vi "Problem 3.vi"(11 "Number to Factor":u64=600851475143) -> (2 "List of Factors":u64[](array[numeric]), 3 "Largest Factor":u64=600851475143)   [LabVIEW 2013, in "Problem 3.lvlib"]
uses:
  Problem 3.lvlib
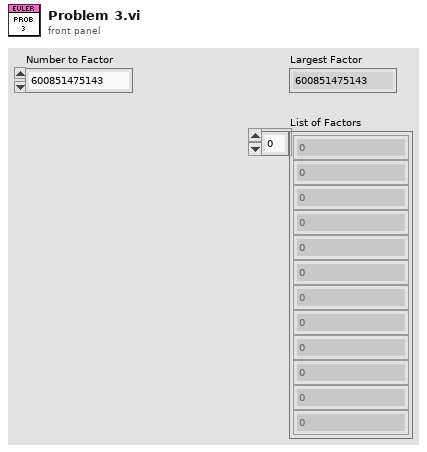
[diagram p1: front panel]
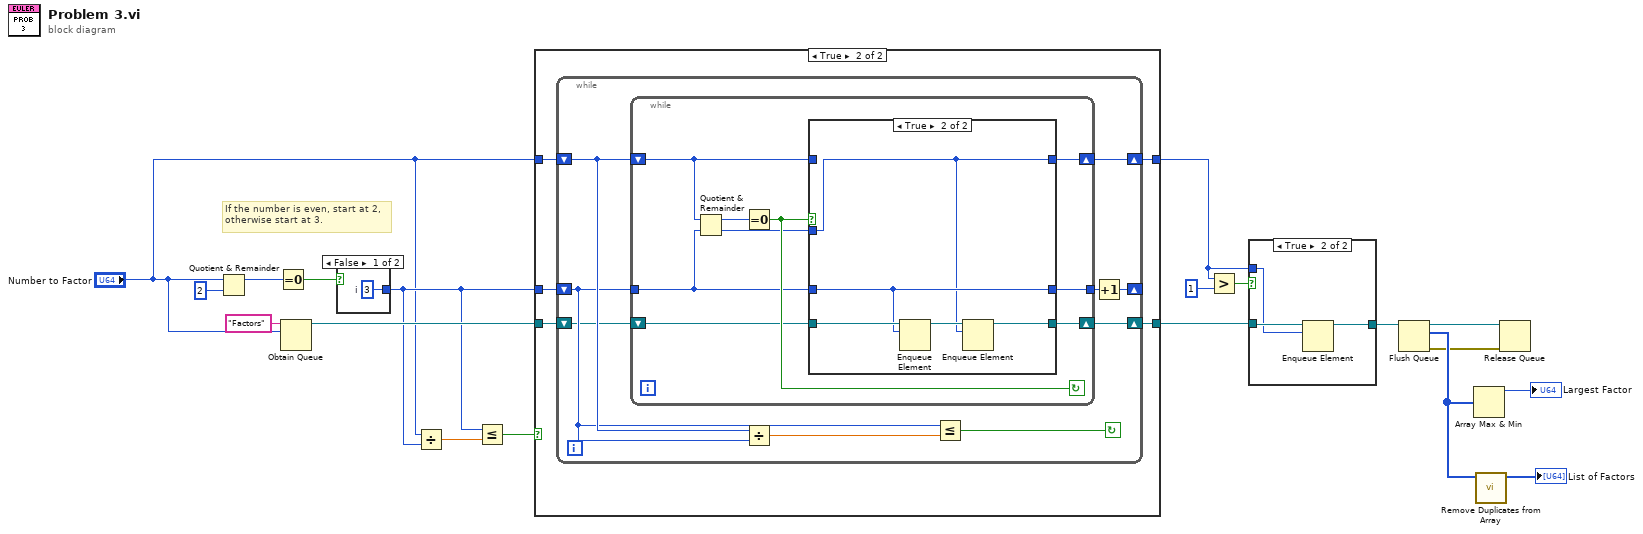
[diagram p0: block diagram]
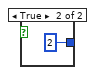
[diagram p5: hidden frame]
diagram:
  # "If the number is even, start at 2,\notherwise start at 3."
  n1 = Quotient & Remainder(x="Number to Factor", y=u64 2) -> (x-y*floor(x/y)=w15:u64)  [unwired: 1 out]
  n2 = Equal To 0?(x=w15) -> (x = 0?=w14:bool)
  n3 = Obtain Queue(name (unnamed)="Factors", element data type="Number to Factor") -> (queue out=w18:refnum<queue>)  [unwired: 3 in, 2 out]
  n4 = case shown="False" w14 {
    tunnel: [w20 u64 2 ("y")] -> w12
    frame False {
      w20 = u64 3  # i
    }
    frame True {
    }
  }
  n5 = Divide(x="Number to Factor", y=w12) -> (x/y=w13:dbl)
  n6 = Less Or Equal?(x=w12, y=w13) -> (x <= y?=w11:bool)
  n7 = case shown="True" w11 {
    tunnel: w18 -> [w23 w28]
    tunnel: [w23 w27] -> w17
    tunnel: "Number to Factor" -> [w22 w26]
    tunnel: w12 -> [_ w25]
    tunnel: [w22 w24] -> w7
    frame False {
    }
    frame True {
      n8 = while {
        shift-right: [w30] -> w27
        shift-left: w28 -> [w32]
        shift-right: [w29] -> _
        shift-left: w25 -> [w34]
        shift-right: [w33] -> w24
        shift-left: w26 -> [w35]
        stop <- w36 continue-if-true
        n9 = while {
          tunnel: w34 -> [w43]
          tunnel: [w39] -> w31
          shift-right: [w38] -> w30
          shift-left: w32 -> [w40]
          shift-right: [w41] -> w33
          shift-left: w35 -> [w44]
          stop <- w45 continue-if-true
          n10 = Quotient & Remainder(x=w44, y=w43) -> (x-y*floor(x/y)=w46:u64, floor(x/y)=w42:u64)
          n11 = Equal To 0?(x=w46) -> (x = 0?=w45:bool)
          n12 = case shown="True" w45 {
            tunnel: w44 -> [w49 _]
            tunnel: w43 -> [w48 w53]
            tunnel: w42 -> [_ w51]
            tunnel: [w49 w51] -> w41
            tunnel: w40 -> [w47 w54]
            tunnel: [w48 w53] -> w39
            tunnel: [w47 w50] -> w38
            frame False {
            }
            frame True {
              n13 = Enqueue Element(queue=w54, element=w53) -> (queue out=w52:refnum<queue>)  [unwired: 2 in, 2 out]
              n14 = Enqueue Element(queue=w52, element=w51) -> (queue out=w50:refnum<queue>)  [unwired: 2 in, 2 out]
            }
          }
        }
        n15 = Divide(x=w35, y=w34) -> (x/y=w37:dbl)
        n16 = Less Or Equal?(x=w34, y=w37) -> (x <= y?=w36:bool)
        n17 = Increment(x=w31) -> (x+1=w29:u64)
      }
    }
  }
  n18 = Greater?(x=w7, y=u64 1) -> (0:w8:bool)
  n19 = case shown="True" w8 {
    tunnel: w17 -> [w55 w58]
    tunnel: w7 -> [_ w57]
    tunnel: [w55 w56] -> w6
    frame False {
    }
    frame True {
      n20 = Enqueue Element(queue=w58, element=w57) -> (queue out=w56:refnum<queue>)  [unwired: 2 in, 2 out]
    }
  }
  n21 = Flush Queue(queue=w6) -> (queue out=w2:refnum<queue>, remaining elements=w4:u64[], error out=w1:errorcluster)  [unwired: 1 in]
  n22 = Array Max & Min(array=w4) -> (max value=→"Largest Factor":u64)  [unwired: 3 out]
  n23 = call "Remove Duplicates from Array.vi"("Array with Duplicates"=w4) -> ("Cleaned Array"=→"List of Factors":u64[])  [unwired: 10 in]
  n24 = Release Queue(queue=w2, error in (no error)=w1) -> ()  [unwired: 1 in, 3 out]
